vi "Request Synchronous Data.vi"   [LabVIEW 2019, in "IObserver.lvlib" / "IObserver.lvclass"]
doc: "DEPRECATED by Request Synchronous Data.vim"
uses:
  <vilib>/gpm_packages/@cs/mva-core/Source/IObserver/IObserver/IObserver.lvclass
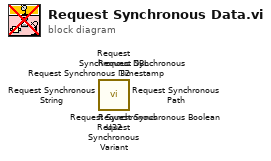
[diagram p0: block diagram]
diagram:
  n1 = call <vilib>:"Request Synchronous U32.vi"() -> ()  [unwired: 8 in, 4 out]
  n2 = call <vilib>:"Request Synchronous Timestamp.vi"() -> ()  [unwired: 8 in, 4 out]
  n3 = call <vilib>:"Request Synchronous String.vi"() -> ()  [unwired: 8 in, 4 out]
  n4 = call <vilib>:"Request Synchronous Path.vi"() -> ()  [unwired: 8 in, 4 out]
  n5 = call <vilib>:"Request Synchronous I32.vi"() -> ()  [unwired: 8 in, 4 out]
  n6 = call <vilib>:"Request Synchronous DBL.vi"() -> ()  [unwired: 8 in, 4 out]
  n7 = call <vilib>:"Request Synchronous Variant.vi"() -> ()  [unwired: 8 in, 4 out]
  n8 = call <vilib>:"Request Synchronous Boolean.vi"() -> ()  [unwired: 8 in, 4 out]
